vi "Delta_Array_Update.vi"(9 "user":i32, 11 "arraylength":i32) -> ()   [LabVIEW 2020]
panel:
  out "user":i32
  out "arraylength":i32
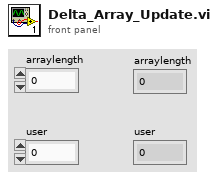
[diagram p1: front panel]
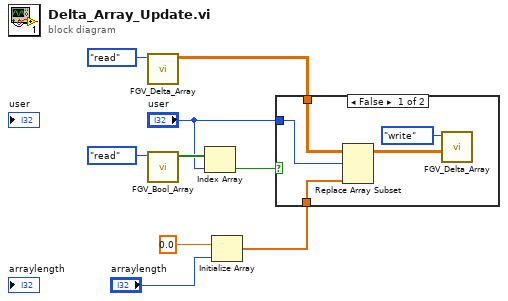
[diagram p0: block diagram]
diagram:
  n1 = call "FGV_Delta_Array.vi"("Enum"=enum16{"read", "write"}."read") -> ("array out"=w4:dbl[][])  [unwired: 10 in]
  n2 = call "FGV_Bool_Array.vi"("Enum"=enum16{"read", "write"}."read") -> ("Array Out"=w7:bool[])  [unwired: 10 in]
  n3 = Index Array(array=w7, index="user") -> (element=w5:bool)
  n4 = Initialize Array(0.0, "arraylength") -> (w2:dbl[])
  n5 = case shown="False" w5 {
    tunnel: w4 -> [w13 _]
    tunnel: w2 -> [w12 _]
    tunnel: "user" -> [w10 _]
    frame False {
      n6 = Replace Array Subset(array=w13, new element=w12, index (row)=w10) -> (w11:dbl[][])  [unwired: 1 in]
      n7 = call "FGV_Delta_Array.vi"("array in"=w11, "Enum"=enum16{"read", "write"}."write") -> ()  [unwired: 9 in, 1 out]
    }
    frame True {
    }
  }
